vi "calculate number of data points and number of snapshots.vi"(8 "Number of CCD bins to use each snapshot":dbl, 9 "Bin width (nm)\n(scan resolution)":dbl[unit], 10 "Start":dbl[unit], 11 "End":dbl[unit]) -> (0 "Number of snapshots required for scan":dbl, 3 "Number of data points in scan":dbl)   [LabVIEW 2023]
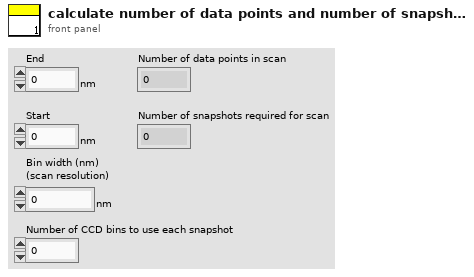
[diagram p1: front panel]
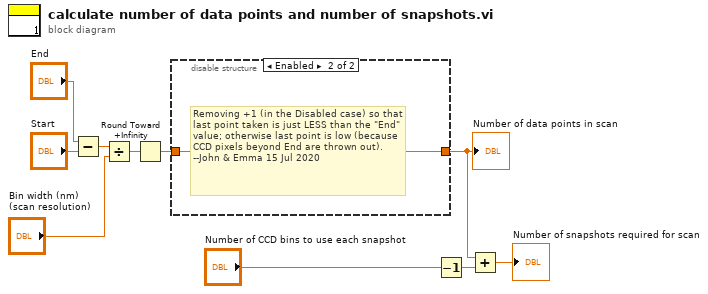
[diagram p0: block diagram]
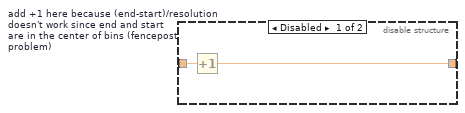
[diagram p2: hidden frame]
diagram:
  n1 = Subtract(x="End", y="Start") -> (x-y=w6:dbl[unit])
  n2 = Divide(x=w6, y="Bin width (nm)\n(scan resolution)") -> (x/y=w9:dbl)
  n3 = Round Toward +Infinity(x=w9) -> (ceil(x): smallest int >= x=w3:dbl)
  n4 = disable-structure shown="Enabled" {
    disable-tunnel: w3 -> [w12 w13]
    disable-tunnel: [w11 w13] -> w1
    frame Disabled {
      n5 = Increment "add +1 here because (end-start)/resolution \ndoesn't work since end and start\nare in the center of bins (fencepost\nproblem)"(x=w12) -> (x+1=w11:dbl)
    }
    frame Enabled {
      # "Removing +1 (in the Disabled case) so that last point taken is just LESS than the \"End\" value; otherwise last point is low (because CCD pixels beyond End are thrown out). \n--John & Emma 15 Jul 2020"
    }
  }
  "Number of data points in scan" <- w1
  n6 = Decrement(x="Number of CCD bins to use each snapshot") -> (x-1=w10:dbl)
  n7 = Add(x=w1, y=w10) -> (x+y=→"Number of snapshots required for scan":dbl)
